vi "Copyright.vi"(10 "error in (no error)":errorcluster) -> (2 "error out":errorcluster, 3 "copyright":string)   [LabVIEW 2014]
doc: "Reads back the copyright"
uses:
  Dependencies/x86/MSC I Process32.dll
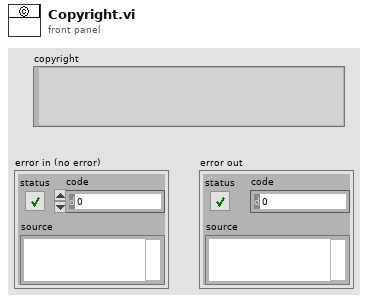
[diagram p1: front panel]
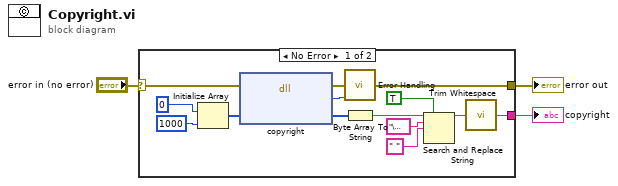
[diagram p0: block diagram]
diagram:
  n1 = case shown="No Error" "error in (no error)" {
    selector: "error in (no error)" -> [w15 w18]
    tunnel: [w14 w18] -> w3
    tunnel: [w4 _] -> w1
    frame No Error {
      n2 = Initialize Array(u8 0, 1000 ("dimension size")) -> (w10:u8[])
      n3 = dll-call lib="C:/Users/MSC/LabVIEW Projekte/LV 2014/MSC I-Process/user.lib/MSC-I Process/Dependencies/x86/MSC I Process*.dll" fn="copyright"(error in=w15, "copyright"=w10) -> (error out=w17:errorcluster, "error"=w16:i32, "copyright"=w13:u8[])  [unwired: 2 in, 1 out]
      n4 = call "Error Handling.vi"("error in (no error)"=w17, "return type"=w16) -> ("error out"=w14:errorcluster)  [unwired: 12 in, 1 out]
      n5 = Byte Array To String(unsigned byte array=w13) -> (string=w5:string)
      n6 = Search and Replace String(replace all?=TRUE ("replace all? (F)"), input string=w5, search string="\u0000", replace string=" " ("replace string (\"\")")) -> (result string=w6:string)  [unwired: 4 in, 3 out]
      n7 = call <vilib>:"Trim Whitespace.vi"("string"=w6) -> ("trimmed string"=w4:string)  [unwired: 1 in]
    }
    frame Error {
    }
  }
  "error out" <- w3
  "copyright" <- w1
